vi "VegaAnalogOutputReadViaUSB6009.vi"() -> ()   [LabVIEW 2017]
uses:
  <vilib>/ptbypt/NI_PtbyPt.lvlib
panel:
  out "mean":dbl format="%0.2f"
  out "data":dynamicdata(graph)
  in  "stop (F)":bool
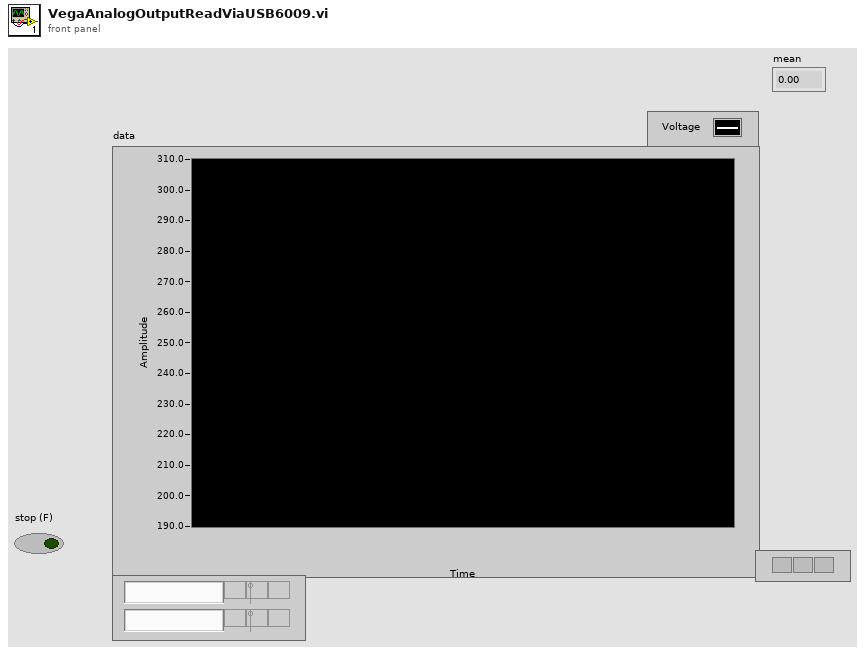
[diagram p1: front panel]
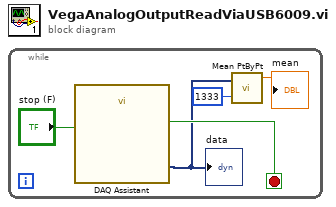
[diagram p0: block diagram]
diagram:
  n1 = while {
    stop <- w4 stop-if-true
    n2 = call "DAQ Assistant"("stop (F)"="stop (F)") -> ("data"=w3:dynamicdata, "stopped"=w4:bool)  [unwired: 15 in, 2 out]
    "data" <- w3
    n3 = call <vilib>:"Mean PtByPt.vi"("x"=w3, "sample length"=1333) -> ("mean"=→"mean":dbl)  [unwired: 2 in, 1 out]
  }
